vi "GetRawAxis.vi"(8 "error in (no error)":errorcluster, 10 "Arduino Resource In":T1={"VISA resource"="", "Board Type"=enum."Uno", "Connection Type"=enum."USB / Serial", "Bytes Per Packet (15)"=15}, 11 "HMC5883L in":refnum<class "HMC5883L.lvclass">) -> (0 "error out":errorcluster, 1 "MagnetometerRaw":cluster{"XAxis":i16, "YAxis":i16, "ZAxis":i16}, 2 "Arduino Resource out":T1={"VISA resource"="", "Board Type"=enum."Uno", "Connection Type"=enum."USB / Serial", "Bytes Per Packet (15)"=15}, 3 "HMC5883L out":refnum<class "HMC5883L.lvclass">)   [LabVIEW 2012, in "HMC5883L.lvclass"]
uses:
  HMC5883L.lvclass
  <vilib>/LabVIEW Interface for Arduino/Type Defs/Board Type.ctl
  <vilib>/LabVIEW Interface for Arduino/LabVIEW Interface for Arduino.lvlib
  <vilib>/LabVIEW Interface for Arduino/Type Defs/Arduino Resource.ctl
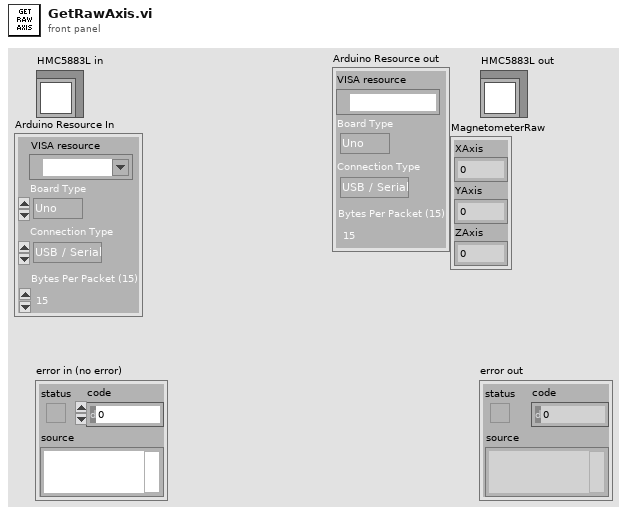
[diagram p1: front panel]
types:
  T1 = typedef "LabVIEW Interface for Arduino.lvlib/Arduino Resource.ctl" = cluster{"VISA resource":refnum<visa-resource-name>, "Board Type":T2, "Connection Type":enum8{"USB / Serial"}, "Bytes Per Packet (15)":u8}
  T2 = typedef "LabVIEW Interface for Arduino.lvlib/Board Type.ctl" = enum16{"Uno", "Dimuelanove w/Atmega 328", "Mega 2560"}
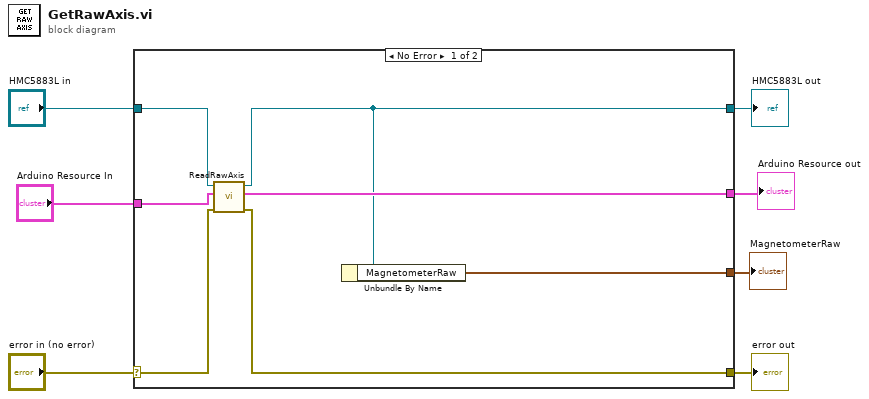
[diagram p0: block diagram]
diagram:
  n1 = case shown="No Error" "error in (no error)" {
    selector: "error in (no error)" -> [w11 w17]
    tunnel: [w10 w17] -> w6
    tunnel: [w9 w16] -> w4
    tunnel: "HMC5883L in" -> [w12 w16]
    tunnel: "Arduino Resource In" -> [w14 w15]
    tunnel: [w13 w15] -> w2
    tunnel: [w8 _] -> w1
    frame No Error {
      n2 = call-dynamic "ReadRawAxis.vi"("error in (no error)"=w11, "Arduino Resource In"=w14, "HMC5883L in"=w12) -> ("error out"=w10:errorcluster, "Arduino Resource out"=w13:T1, "HMC5883L out"=w9:refnum<class "HMC5883L.lvclass">)  [unwired: 6 in]
      n3 = Unbundle By Name(w9) -> ("MagnetometerRaw"=w8:cluster{"XAxis":i16, "YAxis":i16, "ZAxis":i16})
    }
    frame Error {
    }
  }
  "error out" <- w6
  "HMC5883L out" <- w4
  "Arduino Resource out" <- w2
  "MagnetometerRaw" <- w1
